vi "baseline_c.vi"() -> ()   [LabVIEW 2013]
uses:
  project/Baseline/Release/Baseline.dll
panel:
  out "baseline":dbl format="%#_13g"
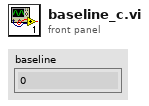
[diagram p1: front panel]
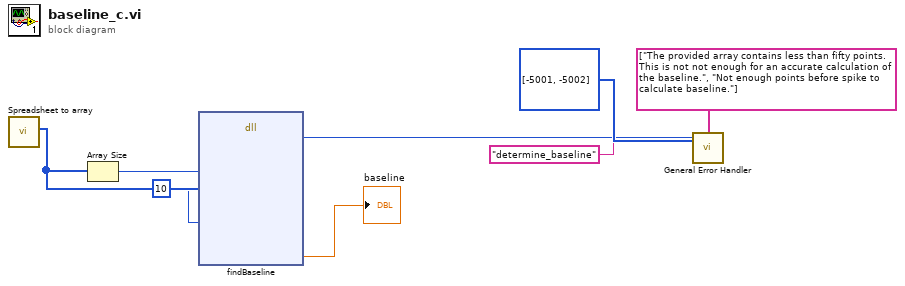
[diagram p0: block diagram]
diagram:
  n1 = call "Spreadsheet to array.vi"() -> ("Array"=w7:u16[])  [unwired: 8 in, 3 out]
  n2 = Array Size(array=w7) -> (size(s)=w8:i32)
  n3 = dll-call lib="C:/Users/SuperUser/Documents/HiSparc/HISPARC_baseline/project/Baseline/Release/Baseline.dll" fn="findBaseline"("array"=w7, "size"=w8, "threshold"=10) -> ("error"=w2:i32, "baseline"=→"baseline":dbl)  [unwired: 13 in, 2 out]
  n4 = call <vilib>:"General Error Handler.vi"("[error code] (0)"=w2, "[user-defined codes]"=i32[] [-5001, -5002], "[user-defined descriptions]"=string[] ["The provided array contains less than fifty points. This is not not enough for an accurate calculation of the baseline.", "Not enough points before spike to calculate baseline."], "[error source] (\" \")"="determine_baseline" ("[error source] (\" \")")) -> ()  [unwired: 7 in, 5 out]
